vi "myPI.vi"(4 "Output limits":cluster{"high":dbl, "low":dbl}, 5 "manual input":dbl, 6 "PID gains":T1, 7 "manual/auto":bool, 8 "dt (s)":dbl, 9 "Integrator in":dbl[](array[numeric]), 10 "setpoint":dbl, 11 "process variable":dbl) -> (1 "Integrator out":dbl[](array[numeric]), 3 "Output":dbl)   [LabVIEW 2020]
panel:
  in  "Anti-windup":bool=TRUE
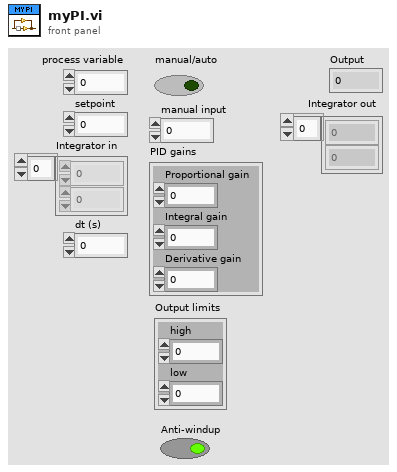
[diagram p1: front panel]
types:
  T1 = cluster{"Proportional gain":dbl, "Integral gain":dbl, "Derivative gain":dbl}
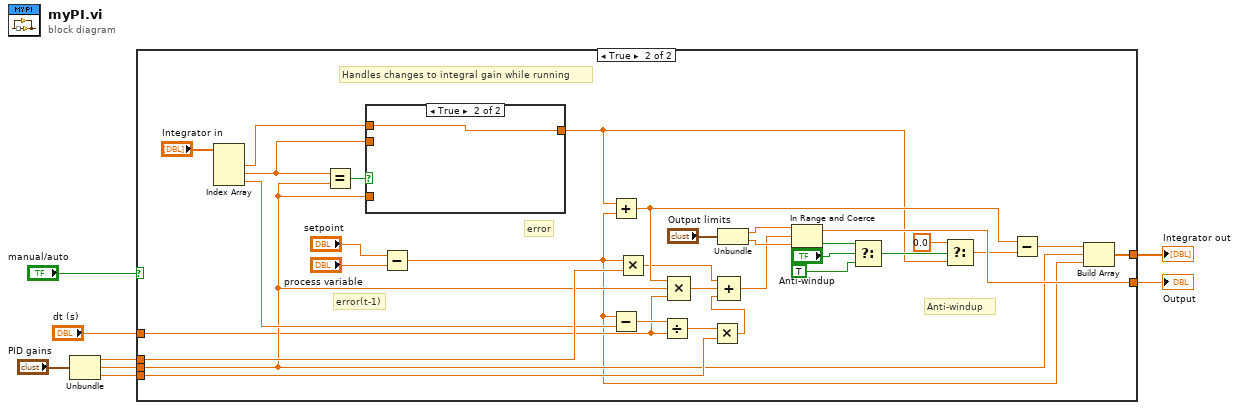
[diagram p0: block diagram]
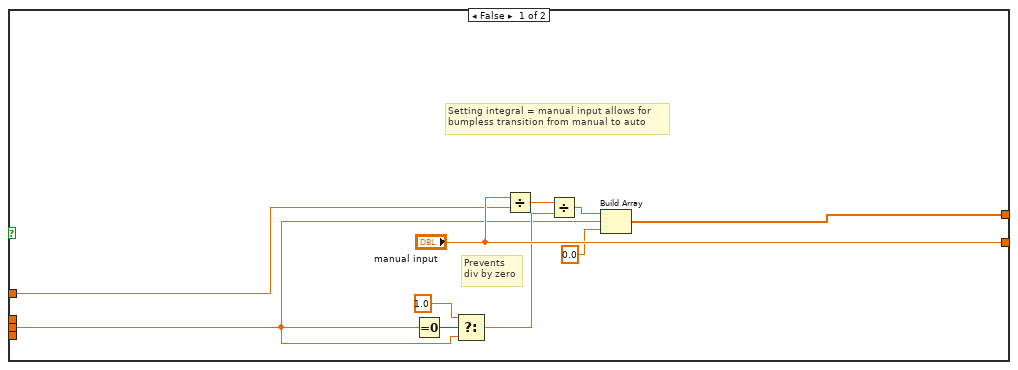
[diagram p2: hidden frame]
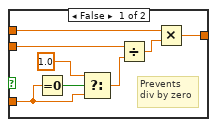
[diagram p3: hidden frame]
diagram:
  n1 = Unbundle("PID gains") -> ("Proportional gain"=w5:dbl, "Integral gain"=w4:dbl, "Derivative gain"=w1:dbl)
  n2 = case shown="True" "manual/auto" {
    tunnel: ["manual input" w50] -> w8
    tunnel: [w10 w40] -> w2
    tunnel: w5 -> [_ w44]
    tunnel: w4 -> [w11 w21]
    tunnel: "dt (s)" -> [w16 w20]
    tunnel: w1 -> [_ w28]
    frame False {
      # "Setting integral = manual input allows for\nbumpless transition from manual to auto"
      # "Prevents\ndiv by zero"
      n3 = Equal To 0?(x=w11) -> (x = 0?=w14:bool)
      n4 = Select(t=1.0, s=w14, f=w11) -> (s? t:f=w13:dbl)
      n5 = Divide(x="manual input", y=w16) -> (x/y=w18:dbl)
      n6 = Divide(x=w18, y=w13) -> (x/y=w12:dbl)
      n7 = Build Array(w12, w11, 0.0 ("element")) -> (w10:dbl[])
    }
    frame True {
      # "error(t-1)"
      # "error"
      # "Handles changes to integral gain while running"
      # "Anti-windup"
      n8 = Index Array(array="Integrator in") -> (element #1=w30:dbl, element #2=w34:dbl, element #3=w25:dbl)  [unwired: 3 in]
      n9 = Equal?(x=w34, y=w21) -> (x = y?=w33:bool)
      n10 = case shown="True" w33 {
        tunnel: w30 -> [w58 w59]
        tunnel: [w57 w59] -> w24
        tunnel: w34 -> [w56 _]
        tunnel: w21 -> [w53 _]
        frame False {
          # "Prevents\ndiv by zero"
          n11 = Equal To 0?(x=w53) -> (x = 0?=w54:bool)
          n12 = Select(t=1.0, s=w54, f=w53) -> (s? t:f=w55:dbl)
          n13 = Divide(x=w56, y=w55) -> (x/y=w51:dbl)
          n14 = Multiply(x=w58, y=w51) -> (x*y=w57:dbl)
        }
        frame True {
        }
      }
      n15 = Subtract(x="setpoint", y="process variable") -> (x-y=w19:dbl)
      n16 = Add(x=w24, y=w19) -> (x+y=w26:dbl)
      n17 = Subtract(x=w19, y=w25) -> (x-y=w31:dbl)
      n18 = Multiply(x=w19, y=w44) -> (x*y=w22:dbl)
      n19 = Divide(x=w31, y=w20) -> (x/y=w29:dbl)
      n20 = Compound Arithmetic op=MULTIPLY(w26, w21, w20) -> (w32:dbl)
      n21 = Multiply(x=w29, y=w28) -> (x*y=w23:dbl)
      n22 = Unbundle("Output limits") -> ("high"=w48:dbl, "low"=w47:dbl)
      n23 = Compound Arithmetic op=ADD(w22, w32, w23) -> (w27:dbl)
      n24 = In Range and Coerce(upper limit=w48, x=w27, lower limit=w47) -> (coerced(x)=w50:dbl, In Range?=w38:bool)
      n25 = Select(t=w38, s="Anti-windup", f=TRUE) -> (s? t:f=w35:bool)
      n26 = Select(t=0.0, s=w35, f=w24) -> (s? t:f=w43:dbl)
      n27 = Subtract(x=w26, y=w43) -> (x-y=w41:dbl)
      n28 = Build Array(w41, w21, w19) -> (w40:dbl[])
    }
  }
  "Output" <- w8
  "Integrator out" <- w2
